vi "delete dublicates in coordinate array.vi"(8 "error in (no error)":errorcluster, 11 "TomoConversion in":refnum<class "TomoConversion.lvclass">) -> (0 "error out":errorcluster, 1 "y coordinate array":string[](array[string]), 2 "x coordinate array":string[](array[string]), 3 "TomoConversion out":refnum<class "TomoConversion.lvclass">)   [LabVIEW 2012, in "TomoConversion.lvclass"]
uses:
  TomoConversion.lvclass
  TomoConversion.lvclass/TomoConversion.ctl
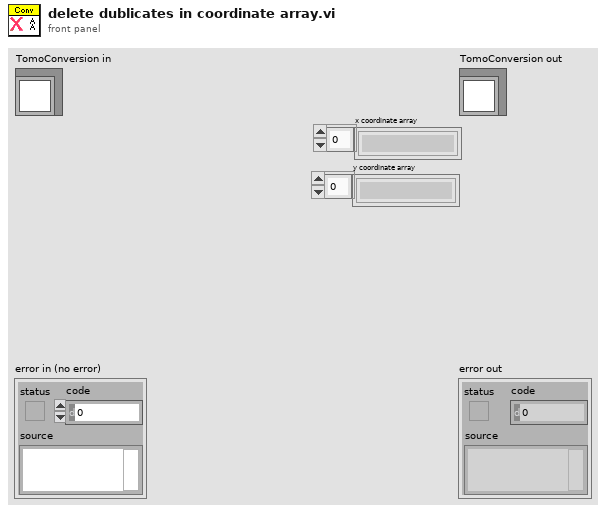
[diagram p1: front panel]
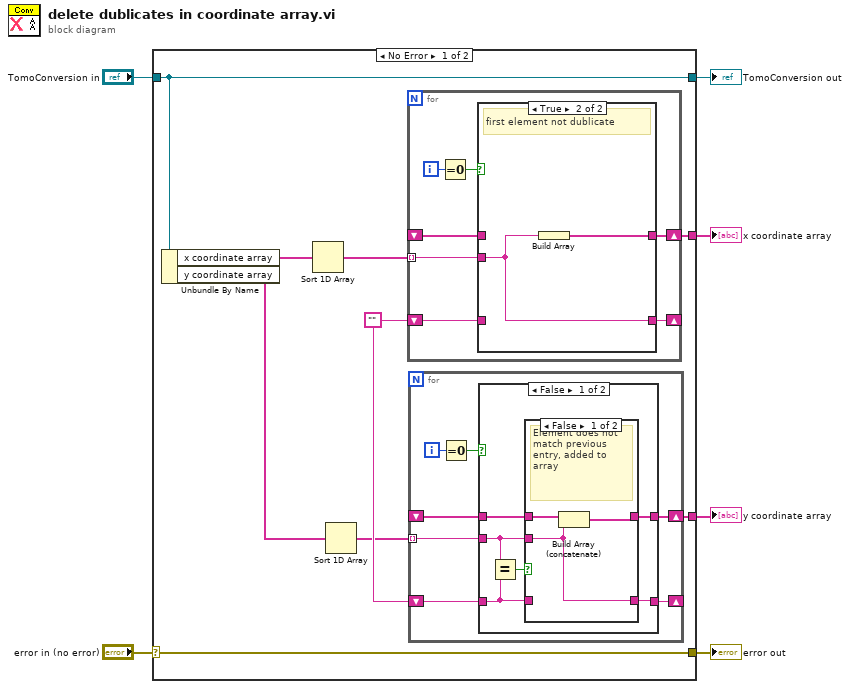
[diagram p0: block diagram]
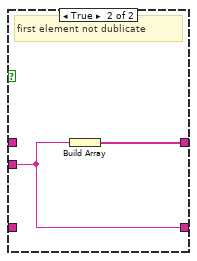
[diagram p3: hidden frame]
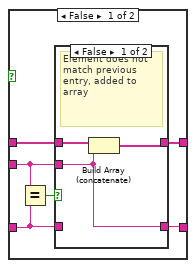
[diagram p4: hidden frame]
diagram:
  n1 = case shown="No Error" "error in (no error)" {
    selector: "error in (no error)" -> [w15 w57]
    tunnel: [w15 w57] -> w5
    tunnel: [w14 w56] -> w3
    tunnel: "TomoConversion in" -> [w14 w56]
    tunnel: [w13 _] -> w2
    tunnel: [w11 _] -> w1
    frame No Error {
      w12 = ""
      n2 = Unbundle By Name(w14) -> ("x coordinate array"=w10:string[], "y coordinate array"=w8:string[])
      n3 = Sort 1D Array(array=w10) -> (sorted array=w9:string[])
      n4 = Sort 1D Array(array=w8) -> (sorted array=w7:string[])
      n5 = for {
        tunnel: w9 -> [w40] mode=indexing
        shift-right: [w38] -> _
        shift-left: w12 -> [w37]
        shift-right: [w39] -> w13
        shift-left: _ -> [w36]
        i -> [w42]
        n6 = Equal To 0?(x=w42) -> (x = 0?=w41:bool)
        n7 = case shown="True" w41 {
          tunnel: w40 -> [w43 w54]
          tunnel: [w44 w55] -> w39
          tunnel: [w46 w54] -> w38
          tunnel: w37 -> [w47 _]
          tunnel: w36 -> [w45 _]
          frame False {
            n8 = Equal?(x=w43, y=w47) -> (x = y?=w48:bool)
            n9 = case shown="False" w48 {
              tunnel: w47 -> [_ w53]
              tunnel: [w49 w53] -> w46
              tunnel: w45 -> [w51 w52]
              tunnel: [w50 w52] -> w44
              tunnel: w43 -> [w49 _]
              frame False {
                # "Element does not match previous entry, added to array"
                n10 = Build Array (concatenate)(w51, w49) -> (w50:string[])
              }
              frame True {
                # "Element matches previous Element, not added"
              }
            }
          }
          frame True {
            # "first element not dublicate"
            n11 = Build Array(w54) -> (w55:string[])
          }
        }
      }
      n12 = for {
        tunnel: w7 -> [w20] mode=indexing
        shift-right: [w18] -> _
        shift-left: w12 -> [w17]
        shift-right: [w19] -> w11
        shift-left: _ -> [w16]
        i -> [w22]
        n13 = Equal To 0?(x=w22) -> (x = 0?=w21:bool)
        n14 = case shown="False" w21 {
          tunnel: w20 -> [w23 w34]
          tunnel: [w24 w35] -> w19
          tunnel: [w26 w34] -> w18
          tunnel: w17 -> [w27 _]
          tunnel: w16 -> [w25 _]
          frame False {
            n15 = Equal?(x=w23, y=w27) -> (x = y?=w28:bool)
            n16 = case shown="False" w28 {
              tunnel: w27 -> [_ w33]
              tunnel: [w29 w33] -> w26
              tunnel: w25 -> [w31 w32]
              tunnel: [w30 w32] -> w24
              tunnel: w23 -> [w29 _]
              frame False {
                # "Element does not match previous entry, added to array"
                n17 = Build Array (concatenate)(w31, w29) -> (w30:string[])
              }
              frame True {
                # "Element matches previous Element, not added"
              }
            }
          }
          frame True {
            # "first element not dublicate"
            n18 = Build Array(w34) -> (w35:string[])
          }
        }
      }
    }
    frame Error {
    }
  }
  "error out" <- w5
  "TomoConversion out" <- w3
  "x coordinate array" <- w2
  "y coordinate array" <- w1
